vi "Execute.vi"(8 "error in":errorcluster, 11 "Cycle State STEP in":refnum<class "Cycle State STEP.lvclass">) -> (0 "error out":errorcluster, 1 "Next Step?":bool, 2 "MSG":string, 3 "Cycle State STEP out":refnum<class "Cycle State STEP.lvclass">)   [LabVIEW 2014, in "Cycle State STEP.lvclass"]
uses:
  Cycle State STEP.lvclass
  reusable/Sequence/STEPS/STEP.lvclass
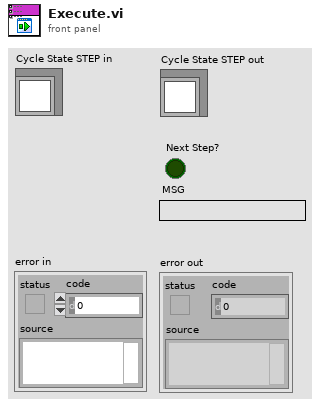
[diagram p1: front panel]
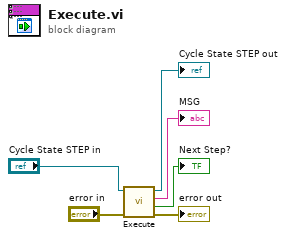
[diagram p0: block diagram]
diagram:
  n1 = call-parent "Execute.vi"("error in"="error in", "STEP in"="Cycle State STEP in") -> ("error out"=→"error out":errorcluster, "Next Step?"=→"Next Step?":bool, "MSG"=→"MSG":string, "STEP out"=→"Cycle State STEP out":refnum<class "Cycle State STEP.lvclass">)  [unwired: 6 in]
